vi "Write CAN FIFO.vi"(4 "T_Out":u64, 6 "T0":u64, 8 "error in (no error)":errorcluster, 9 "Timeout (ms)":i32, 10 "Data":T1 {"payload" format="%x"; "identifier" format="%x"}, 11 "CIFTag in":refnum<class "CIFFifoCAN.lvclass">) -> (0 "error out":errorcluster, 1 "timed out?":bool, 3 "CIFTag out":refnum<class "CIFFifoCAN.lvclass">)   [LabVIEW 2021, in "CIFFifoCAN.lvclass"]
uses:
  CIFFifoCAN.lvclass
  D:/dev/CIF-LVCore/src/Channels/CIFTag/CIFTag/CIFTag.lvclass
  ChannelRegistrar/typedef/Datatype CAN.ctl
  CIFFifoCAN.lvclass/CIFFifoCAN.ctl
  CIFFIFO/CIFfifo.lvclass/CIFfifo.ctl
  CIFTag/CIFTag.lvclass/CIFTag.ctl
  CIFFIFO/Accessors/Read Length.vi
  <vilib>/CIFChannels/SubVIs/Get dll Path.vi
  CIFFIFO/Utilities/Update Header.vi
  ChannelCommon/Utilities/Flatten Header.vi
  SubVIs/Flatten.vi/e2488641-f297-4923-bbd0-3c2628a14485.vi
  CIFFIFO/Accessors/Write T0.vi
  CIFFIFO/Accessors/Write T_Out.vi
  CIFFIFO/Accessors/Write Payload Length.vi
  CIFFIFO/Accessors/Read Header.vi
  CIFFIFO/Accessors/Write Header.vi
  CIFUtilities/CIFClocks/SubVIs/Add Error.vi
  SubVIs/Flatten.vi/e2488641-f297-4923-bbd0-3c2628a14485.vi/c28b0ead-42ad-4072-80a2-aca7f2bd7ce3.vi
  CIFCore/Common/Utilities/Append Error Location.vi
  ChannelCommon/Utilities/Update Time.vi
  CIFTag/CIFTag.lvclass
  <vilib>/CIFChannels/CIFChannelCore.lvlib
  CIFFIFO/CIFfifo.lvclass
  ChannelRegistrar/ChannelRegistrar.lvlib
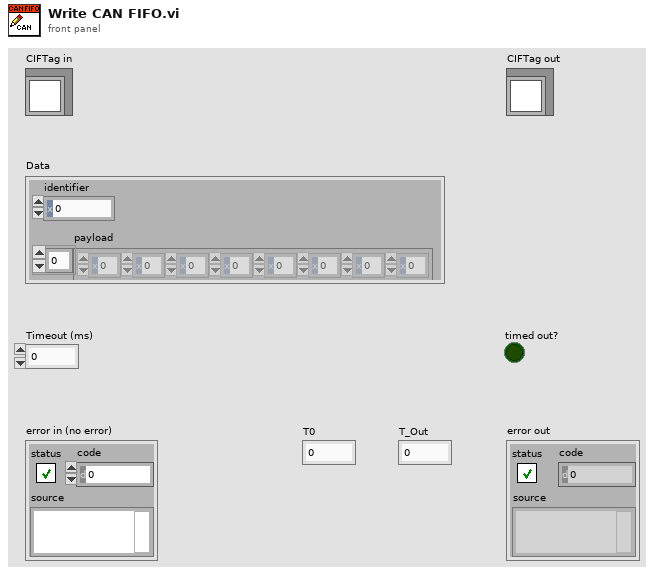
[diagram p1: front panel]
types:
  T1 = typedef "ChannelRegistrar.lvlib/Datatype CAN.ctl" = cluster{"payload":u8[], "identifier":u32}
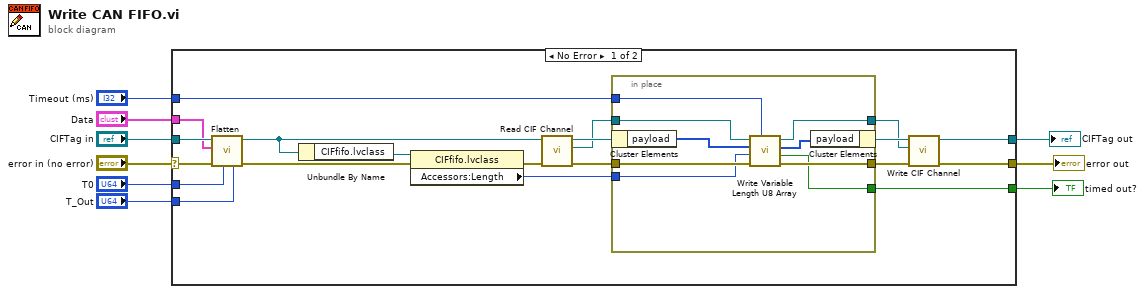
[diagram p0: block diagram]
diagram:
  n1 = case shown="No Error" "error in (no error)" {
    selector: "error in (no error)" -> [w13 w40]
    tunnel: [w20 w40] -> w8
    tunnel: [w25 w39] -> w6
    tunnel: "CIFTag in" -> [w17 w39]
    tunnel: [w29 _] -> w5
    tunnel: "Timeout (ms)" -> [w21 _]
    tunnel: "T_Out" -> [w11 _]
    tunnel: "T0" -> [w12 _]
    tunnel: "Data" -> [w14 _]
    frame No Error {
      n2 = call "Flatten.vi"("T_Out"=w11, "T0"=w12, "error in (no error)"=w13, "Data"=w14, "CIFTag in"=w17) -> ("error out"=w15:errorcluster, "CIFTag out"=w16:refnum<class "CIFFifoCAN.lvclass">)  [unwired: 5 in]
      n3 = Unbundle By Name(w16) -> ("CIFfifo.lvclass"=w19:refnum<class "CIFfifo.lvclass">)
      n4 = property class="CIFfifo.lvclass"(reference=w19, error in=w15) -> (error out=w18:errorcluster, "Accessors:Length"=w10:u64)  [unwired: 1 out]
      n5 = call "Read CIF Channel.vi"("error in (no error)"=w18, "CIFTag in"=w16) -> ("error out"=w27:errorcluster, "CIF Channel"=w23:refnum<k21>, "CIFTag out"=w28:refnum<class "CIFFifoCAN.lvclass">)  [unwired: 7 in]
      n6 = in-place {
        in-place-border: w27 -> [w38]
        in-place-border: [w37] -> w24
        in-place-border: [w36] -> w29
        in-place-border: w23 -> [w35]
        in-place-border: [w34] -> w22
        in-place-border: w21 -> [w33]
        in-place-border: w10 -> [w31]
        n7 = in-place-cluster #1(w28) -> ("payload"=w32:u8[])
        n8 = call <vilib>:"Write Variable Length U8 Array.vi"("Timeout (ms)"=w33, "error in"=w38, "numElements"=w31, "U8 Array in"=w32, "CIF Channel in"=w35) -> ("error out"=w37:errorcluster, "Timed out?"=w36:bool, "U8 Array out"=w30:u8[], "CIF Channel out"=w34:refnum<k21>)  [unwired: 3 in]
        n9 = in-place-cluster #1("payload"=w30) -> (w26:refnum<class "CIFFifoCAN.lvclass">)
      }
      n10 = call "Write CIF Channel.vi"("error in (no error)"=w24, "CIF Channel"=w22, "CIFTag in"=w26) -> ("error out"=w20:errorcluster, "CIFTag out"=w25:refnum<class "CIFFifoCAN.lvclass">)  [unwired: 7 in]
    }
    frame Error {
    }
  }
  "error out" <- w8
  "CIFTag out" <- w6
  "timed out?" <- w5
